vi "Save gate sweep.vi"(4 "seconds since 1Jan1904":timestamp, 5 "Numeric 2":i32, 6 "Array":dbl[](array[numeric]), 7 "Array 2":dbl[](array[numeric]), 8 "error in (no error)":errorcluster, 9 "Boolean":bool, 10 "Numeric":dbl, 11 "Refnum in":refnum<k34>) -> (0 "error out":errorcluster, 3 "Refnum out":refnum<k34>)   [LabVIEW 2017]
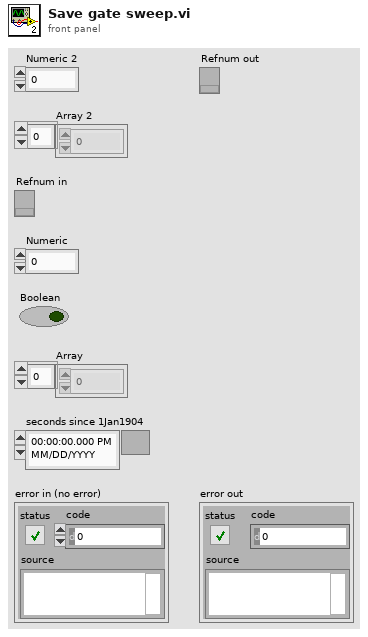
[diagram p1: front panel]
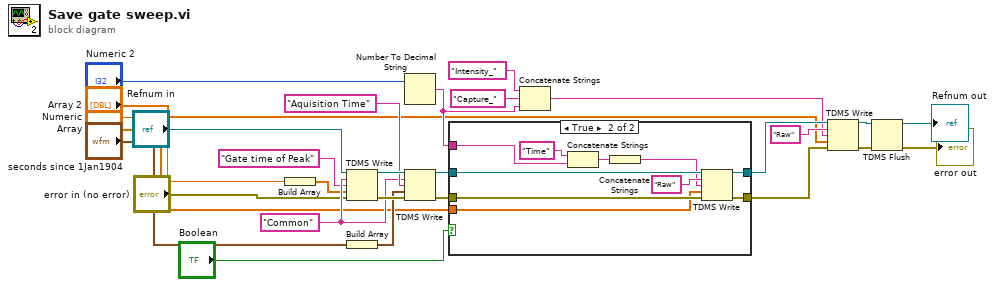
[diagram p0: block diagram]
diagram:
  w16 = "Common" ("group name in (Untitled)")
  n1 = Build Array("Numeric") -> (w7:dbl[])
  n2 = TDMS Write(0:"Refnum in", 5:w16, 7:"Gate time of Peak", 9:w7, 11:"error in (no error)") -> (4:w22:refnum<k34>, 15:w23:errorcluster)  [unwired: 1 in, 2 out]
  n3 = Build Array("seconds since 1Jan1904") -> (w18:timestamp[])
  n4 = Number To Decimal String(number="Numeric 2") -> (decimal integer string=w28:string)  [unwired: 1 in]
  n5 = TDMS Write(0:w22, 5:w16, 7:"Aquisition Time", 9:w18, 11:w23) -> (4:w20:refnum<k34>, 15:w21:errorcluster)  [unwired: 1 in, 2 out]
  n6 = case shown="True" "Boolean" {
    tunnel: w20 -> [w30 w40]
    tunnel: w21 -> [w29 w39]
    tunnel: [w30 w38] -> w13
    tunnel: [w29 w37] -> w12
    tunnel: "Array" -> [_ w34]
    tunnel: w28 -> [_ w31]
    frame False {
    }
    frame True {
      n7 = Concatenate Strings("Time" ("string"), w31) -> (w33:string)
      n8 = Concatenate Strings(w33) -> (w35:string)
      n9 = TDMS Write(0:w40, 5:"Raw" ("group name in (Untitled)"), 7:w35, 9:w34, 11:w39) -> (4:w38:refnum<k34>, 15:w37:errorcluster)  [unwired: 1 in, 2 out]
    }
  }
  n10 = Concatenate Strings("Intensity_" ("group name in (Untitled)"), "Capture_" ("string"), w28) -> (w10:string)
  n11 = TDMS Write(0:w13, 5:"Raw" ("group name in (Untitled)"), 7:w10, 9:"Array 2", 11:w12) -> (4:w24:refnum<k34>, 15:w25:errorcluster)  [unwired: 1 in, 2 out]
  n12 = TDMS Flush(4:w25, 7:w24) -> (0:→"error out":errorcluster, 3:→"Refnum out":refnum<k34>)
